vi "DriveTalonModeOverride.vi"(5 "Coast":bool, 7 "Brake":bool) -> ()   [LabVIEW 2014]
uses:
  <vilib>/Rock Robotics/WPI/CAN/TalonSRX/WPI_CANTalonSRX_BrakeOverride.ctl
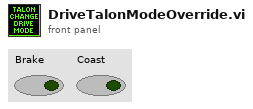
[diagram p1: front panel]
types:
  T1 = typedef "WPI_CANTalonSRX_BrakeOverride.ctl" = enum8{"No Override", "Override to Coast", "Override to Brake"}
  T2 = typedef "WPI_MotorControlDeviceRef.ctl" = cluster{"DeviceStatus":errorcluster, "Type":T3, "PWM":cluster{"Controller":T4, "PWM Channel":T5, "DeadBand":T6}, "CAN":cluster{"Device Number":u8, "Control Mode":T7, "Semaphore":T8, "Max Vout":dbl, "TalonSRX Control Mode":T9}, "Invert":bool, "TransformRef":T10, "InvTransformRef":T10}
  T3 = typedef "WPI_MotorControlType.ctl" = enum16{"PWM", "CAN", "CANTalonSRX"}
  T4 = typedef "FPGA_TypedefDigitalModule.ctl" = enum16{"Controller 1"}
  T5 = typedef "FPGA_DIOPWMChannel.ctl" = enum8{"PWM 0", "PWM 1", "PWM 2", "PWM 3", "PWM 4", "PWM 5", "PWM 6", "PWM 7", "PWM 8", "PWM 9", "PWM MXP 0", "PWM MXP 1", "PWM MXP 2", "PWM MXP 3", "PWM MXP 4", "PWM MXP 5", "PWM MXP 6", "PWM MXP 7", "PWM MXP 8", "PWM MXP 9", "Invalid"}
  T6 = typedef "WPI_PWMDeadband.ctl" = cluster{"Name":string, "maxPositivePwm":i32, "minPositivePwm":i32, "centerPwm":i32, "maxNegativePwm":i32, "minNegativePwm":i32, "angularRange":u16}
  T7 = typedef "WPI_CANJaguar_ControlMode.ctl" = enum8{"Percent VBus", "Current", "Speed", "Position", "Voltage"}
  T8 = typedef "Semaphore RefNum" = refnum<k1>
  T9 = typedef "WPI_CANTalonSRX_APIControlMode.ctl" = enum8{"Percent VBus", "Speed", "Position", "Slave", "Unchanged / Invalid"}
  T10 = typedef "WPI_PWMTransform_ConPane.ctl" = refnum<vi>
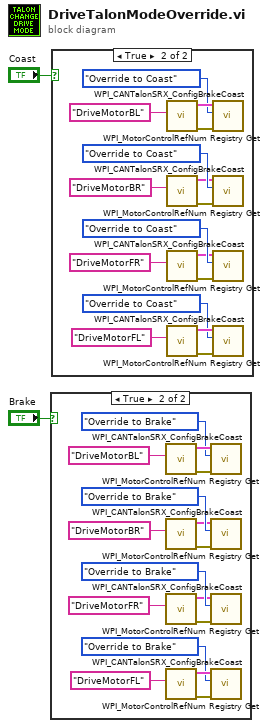
[diagram p0: block diagram]
diagram:
  n1 = case shown="True" "Brake" {
    frame False {
    }
    frame True {
      n2 = call <vilib>:"WPI_MotorControlRefNum Registry Get.vi"("refnum name"="DriveMotorBL") -> ("error out"=w9:errorcluster, "MotorControlDevRef"=w8:T2)  [unwired: 9 in]
      n3 = call <vilib>:"WPI_MotorControlRefNum Registry Get.vi"("refnum name"="DriveMotorBR") -> ("error out"=w4:errorcluster, "MotorControlDevRef"=w5:T2)  [unwired: 9 in]
      n4 = call <vilib>:"WPI_MotorControlRefNum Registry Get.vi"("refnum name"="DriveMotorFR") -> ("error out"=w12:errorcluster, "MotorControlDevRef"=w13:T2)  [unwired: 9 in]
      n5 = call <vilib>:"WPI_MotorControlRefNum Registry Get.vi"("refnum name"="DriveMotorFL") -> ("error out"=w17:errorcluster, "MotorControlDevRef"=w16:T2)  [unwired: 9 in]
      n6 = call <vilib>:"WPI_CANTalonSRX_ConfigBrakeCoast.vi"("error in (no error)"=w9, "Brake / Coast Mode"=WPI_CANTalonSRX_BrakeOverride."Override to Brake", "CAN Talon SRX Ref"=w8) -> ()  [unwired: 7 in, 2 out]
      n7 = call <vilib>:"WPI_CANTalonSRX_ConfigBrakeCoast.vi"("error in (no error)"=w4, "Brake / Coast Mode"=WPI_CANTalonSRX_BrakeOverride."Override to Brake", "CAN Talon SRX Ref"=w5) -> ()  [unwired: 7 in, 2 out]
      n8 = call <vilib>:"WPI_CANTalonSRX_ConfigBrakeCoast.vi"("error in (no error)"=w12, "Brake / Coast Mode"=WPI_CANTalonSRX_BrakeOverride."Override to Brake", "CAN Talon SRX Ref"=w13) -> ()  [unwired: 7 in, 2 out]
      n9 = call <vilib>:"WPI_CANTalonSRX_ConfigBrakeCoast.vi"("error in (no error)"=w17, "Brake / Coast Mode"=WPI_CANTalonSRX_BrakeOverride."Override to Brake", "CAN Talon SRX Ref"=w16) -> ()  [unwired: 7 in, 2 out]
    }
  }
  n10 = case shown="True" "Coast" {
    frame False {
    }
    frame True {
      n11 = call <vilib>:"WPI_MotorControlRefNum Registry Get.vi"("refnum name"="DriveMotorBL") -> ("error out"=w25:errorcluster, "MotorControlDevRef"=w24:T2)  [unwired: 9 in]
      n12 = call <vilib>:"WPI_MotorControlRefNum Registry Get.vi"("refnum name"="DriveMotorBR") -> ("error out"=w20:errorcluster, "MotorControlDevRef"=w21:T2)  [unwired: 9 in]
      n13 = call <vilib>:"WPI_MotorControlRefNum Registry Get.vi"("refnum name"="DriveMotorFR") -> ("error out"=w28:errorcluster, "MotorControlDevRef"=w29:T2)  [unwired: 9 in]
      n14 = call <vilib>:"WPI_MotorControlRefNum Registry Get.vi"("refnum name"="DriveMotorFL") -> ("error out"=w33:errorcluster, "MotorControlDevRef"=w32:T2)  [unwired: 9 in]
      n15 = call <vilib>:"WPI_CANTalonSRX_ConfigBrakeCoast.vi"("error in (no error)"=w25, "Brake / Coast Mode"=WPI_CANTalonSRX_BrakeOverride."Override to Coast", "CAN Talon SRX Ref"=w24) -> ()  [unwired: 7 in, 2 out]
      n16 = call <vilib>:"WPI_CANTalonSRX_ConfigBrakeCoast.vi"("error in (no error)"=w20, "Brake / Coast Mode"=WPI_CANTalonSRX_BrakeOverride."Override to Coast", "CAN Talon SRX Ref"=w21) -> ()  [unwired: 7 in, 2 out]
      n17 = call <vilib>:"WPI_CANTalonSRX_ConfigBrakeCoast.vi"("error in (no error)"=w28, "Brake / Coast Mode"=WPI_CANTalonSRX_BrakeOverride."Override to Coast", "CAN Talon SRX Ref"=w29) -> ()  [unwired: 7 in, 2 out]
      n18 = call <vilib>:"WPI_CANTalonSRX_ConfigBrakeCoast.vi"("error in (no error)"=w33, "Brake / Coast Mode"=WPI_CANTalonSRX_BrakeOverride."Override to Coast", "CAN Talon SRX Ref"=w32) -> ()  [unwired: 7 in, 2 out]
    }
  }
